vi "Build Action.vi"(6 "Build number":u32, 7 "CmdLineArgs":T1={"BuildNumber"=0, "Error"=path "", "Running"=path "", "Workspace"=path "", "Job"="", "MClog"=path "", "BuildLog"=path "", "Copy Built"=TRUE, "SourceVer"="", "MaxBuildVer"=""}, 8 "error in":errorcluster, 9 "VerMismatch?":bool, 10 "Build Spec Info":T2, 11 "App Builder VI in":refnum<vi>) -> (0 "error out":errorcluster, 3 "App Builder VI out":refnum<vi>)   [LabVIEW 2010]
uses:
  Types/Job Type.ctl
  Types/Task Info.ctl
  Types/Command Line Args.ctl
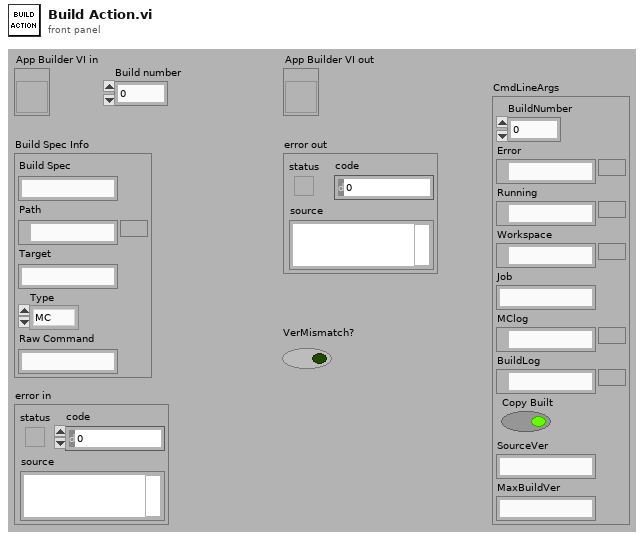
[diagram p1: front panel]
types:
  T1 = typedef "Command Line Args.ctl" = cluster{"BuildNumber":u32, "Error":path, "Running":path, "Workspace":path, "Job":string, "MClog":path, "BuildLog":path, "Copy Built":bool, "SourceVer":string, "MaxBuildVer":string}
  T2 = typedef "Task Info.ctl" = cluster{"Build Spec":string, "Path":path, "Target":string, "Type":T3, "Raw Command":string}
  T3 = typedef "Job Type.ctl" = enum16{"MC", "NOP", "VI", "Build", "VIP", "VIPB", "VIA"}
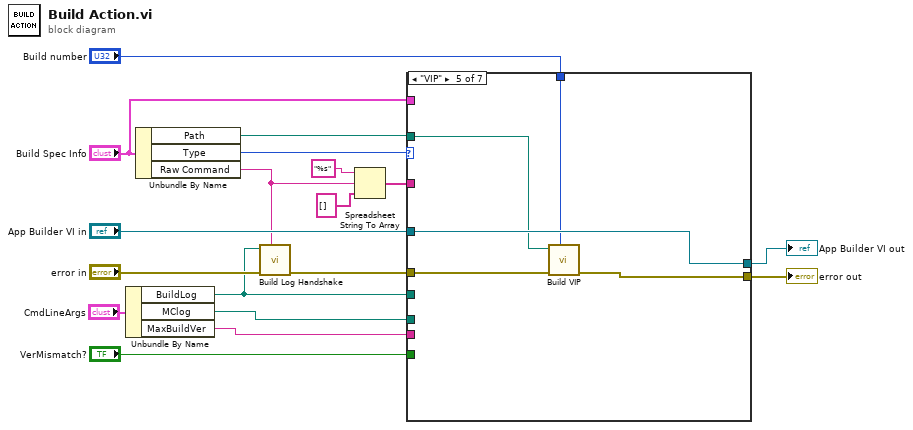
[diagram p0: block diagram]
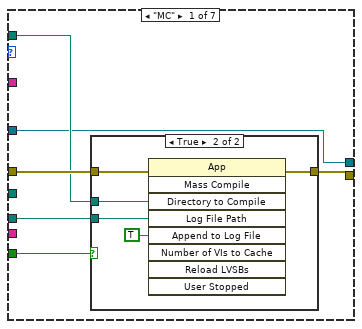
[diagram p2: hidden frame]
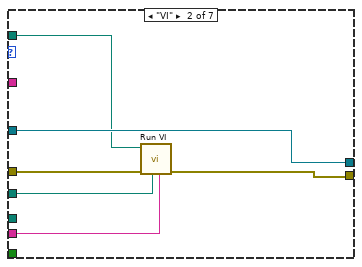
[diagram p4: hidden frame]
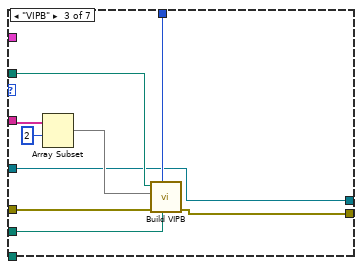
[diagram p5: hidden frame]
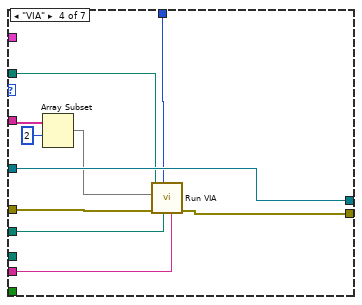
[diagram p6: hidden frame]
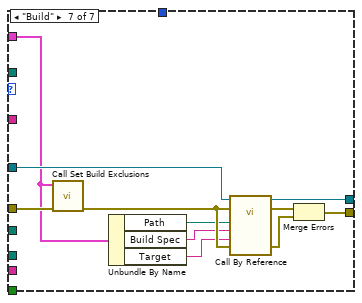
[diagram p8: hidden frame]
diagram:
  n1 = Unbundle By Name("CmdLineArgs") -> ("BuildLog"=w7:path, "MClog"=w6:path, "MaxBuildVer"=w5:string)
  n2 = Unbundle By Name("Build Spec Info") -> ("Path"=w16:path, "Type"=w14:T3, "Raw Command"=w2:string)
  n3 = call "Build Log Handshake.vi"("Command"=w2, "error in (no error)"="error in", "BuildLog"=w7) -> ("error out"=w11:errorcluster)  [unwired: 8 in]
  n4 = Spreadsheet String To Array(format string="%s", spreadsheet string=w2, array type (2D Dbl)=string[] []) -> (array=w1:string[])  [unwired: 1 in]
  n5 = case shown="\"VIP\"" w14 {
    tunnel: [w20 w36 w37 w53 w60 w62 w73] -> w18
    tunnel: [w21 w34 w44 w51 w58 w61 w72] -> w17
    tunnel: w11 -> [w24 w35 w45 w52 w59 w61 w68]
    tunnel: w16 -> [w23 w33 w40 w49 w57 _ _]
    tunnel: "App Builder VI in" -> [w20 w36 w37 w53 w60 w62 w69]
    tunnel: w6 -> [w22 _ _ _ _ _ _]
    tunnel: "VerMismatch?" -> [w19 _ _ _ _ _ _]
    tunnel: "Build Spec Info" -> [_ _ _ _ _ _ w63]
    tunnel: "Build number" -> [_ _ w39 w47 w56 _ _]
    tunnel: w7 -> [_ w32 w38 w50 _ _ _]
    tunnel: w5 -> [_ w31 _ w46 _ _ _]
    tunnel: w1 -> [_ _ w43 w55 _ _ _]
    frame "MC" {
      n6 = case shown="True" w19 {
        tunnel: w24 -> [w25 w30]
        tunnel: w23 -> [_ w29]
        tunnel: w22 -> [_ w28]
        tunnel: [w25 w26] -> w21
        frame False {
        }
        frame True {
          n7 = invoke class="App" method="Mass Compile"(error in=w30, "Directory to Compile"=w29, "Log File Path"=w28, "Append to Log File"=TRUE) -> (error out=w26:errorcluster)  [unwired: 5 in, 8 out]
        }
      }
    }
    frame "VI" {
      n8 = call "Run VI.vi"("MaxBuildVer"=w31, "Buildlog"=w32, "error in (no error)"=w35, "VI Path"=w33) -> ("error out"=w34:errorcluster)  [unwired: 7 in]
    }
    frame "VIPB" {
      n9 = Array Subset(array=w43, index=2) -> (w41:string[])  [unwired: 1 in]
      n10 = call "Build VIPB.vi"("Buildlog"=w38, "Build number"=w39, "error in"=w45, "args"=w41, "VIP Path"=w40) -> ("error out"=w44:errorcluster)  [unwired: 6 in]
    }
    frame "VIA" {
      n11 = Array Subset(array=w55, index=2) -> (w48:string[])  [unwired: 1 in]
      n12 = call "Run VIA.vi"("MaxBuildVer"=w46, "Buildlog"=w50, "Build number"=w47, "error in (no error)"=w52, "args"=w48, "VI Path"=w49) -> ("error out"=w51:errorcluster)  [unwired: 5 in]
    }
    frame "VIP" {
      n13 = call "Build VIP.vi"("Build number"=w56, "error in (no error)"=w59, "VIP Path"=w57) -> ("error out"=w58:errorcluster)  [unwired: 8 in]
    }
    frame "NOP" {
    }
    frame "Build" {
      n14 = call "Call Set Build Exclusions.vi"("error in (no error)"=w68, "Build Spec Info in"=w63) -> ("error out"=w67:errorcluster)  [unwired: 9 in]
      n15 = Unbundle By Name(w63) -> ("Path"=w66:path, "Build Spec"=w65:string, "Target"=w64:string)
      n16 = call-by-ref "?"(reference=w69, error in=w67, 8:"error in (no error)"=w67, "Name of target (My Computer)"=w64, "Name of build specification (if empty: build all)"=w65, "Path to project"=w66) -> (reference out=w73:refnum<vi>, error out=w70:errorcluster, 0:"error out"=w71:errorcluster)  [unwired: 6 in, 1 out]
      n17 = Merge Errors(w70, w71) -> (w72:errorcluster)
    }
  }
  "App Builder VI out" <- w18
  "error out" <- w17
